vi "Move Rotations (SubVI).vi"(8 "Reset":bool, 9 "SwitchValue":bool, 10 "Trigger":i32=4, 11 "Direction":T1=enum."Forward") -> (1 "Rotations":i32, 2 "RelayOutput":T1)   [LabVIEW 2013]
uses:
  <vilib>/Rock Robotics/WPI/Relay/WPI_RelayValue.ctl
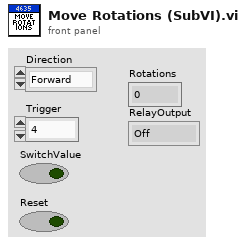
[diagram p1: front panel]
types:
  T1 = typedef "WPI_RelayValue.ctl" = enum16{"Off", "On", "Forward", "Reverse"}
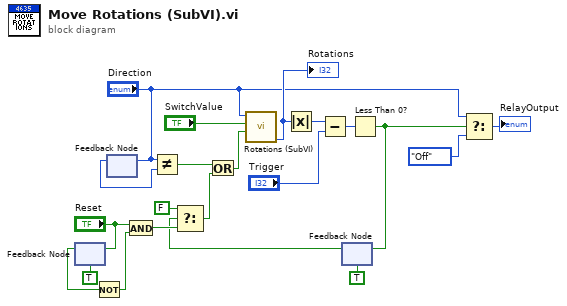
[diagram p0: block diagram]
diagram:
  n1 = feedback #1(TRUE) -> (w8:bool)
  n2 = feedback-in #1("Reset") -> ()
  n3 = Not(x=w8) -> (.not. x?=w9:bool)
  n4 = feedback #2() -> (w12:T1)  [unwired: 1 in]
  n5 = feedback-in #2("Direction") -> ()
  n6 = And(x="Reset", y=w9) -> (x .and. y?=w11:bool)
  n7 = Not Equal?(x="Direction", y=w12) -> (x != y?=w15:bool)
  n8 = feedback #3(TRUE) -> (w2:bool)
  n9 = Select(t=FALSE, s=w2, f=w11) -> (s? t:f=w14:bool)
  n10 = Or(x=w15, y=w14) -> (x .or. y?=w16:bool)
  n11 = call "Rotations (SubVI).vi"("RelayValue"="Direction", "SwitchValue"="SwitchValue", "Reset"=w16) -> ("Rotations"=w19:i32)  [unwired: 7 in]
  "Rotations" <- w19
  n12 = Absolute Value(x=w19) -> (abs(x)=w5:i32)
  n13 = Subtract(x=w5, y="Trigger") -> (x-y=w3:i32)
  n14 = Less Than 0?(x=w3) -> (x < 0?=w1:bool)
  n15 = feedback-in #3(w1) -> ()
  n16 = Select(t="Direction", s=w1, f=WPI_RelayValue."Off" ("RelayValue")) -> (s? t:f=→"RelayOutput":T1)
